vi "CompVisionUtil_EstimateFieldToRobot.vi"(4 "CameraToRobot":T1={"TRANSLATION"={"X"=0.0, "Y"=0.0}, "ROTATION"={"VALUE"=0.0, "COS"=1.0, "SIN"=0.0}, "xF"=FALSE} {"ROTATION"."SIN" format="%13.4f"; "ROTATION"."COS" format="%13.4f"; "ROTATION"."VALUE" format="%13.4f"; "TRANSLATION"."Y" format="%14.3f"; "TRANSLATION"."X" format="%14.3f"}, 5 "cameraHeight_Meters":dbl, 6 "FieldToTarget":T4={"TRANSLATION"={"X"=0.0, "Y"=0.0}, "ROTATION"={"VALUE"=0.0, "COS"=1.0, "SIN"=0.0}} {"ROTATION"."SIN" format="%13.4f"; "ROTATION"."COS" format="%13.4f"; "ROTATION"."VALUE" format="%13.4f"; "TRANSLATION"."Y" format="%14.3f"; "TRANSLATION"."X" format="%14.3f"}, 7 "targetHeight_Meters":dbl, 8 "GyroAngle":T3={"VALUE"=0.0, "COS"=1.0, "SIN"=0.0} {"SIN" format="%13.4f"; "COS" format="%13.4f"; "VALUE" format="%13.4f"}, 9 "TargetYaw":T3={"VALUE"=0.0, "COS"=1.0, "SIN"=0.0} {"SIN" format="%13.4f"; "COS" format="%13.4f"; "VALUE" format="%13.4f"}, 10 "targetPitch_Radians":dbl, 11 "cameraPitch_Radians":dbl) -> (3 "EstimateFieldToRobot":T4={"TRANSLATION"={"X"=0.0, "Y"=0.0}, "ROTATION"={"VALUE"=0.0, "COS"=1.0, "SIN"=0.0}} {"ROTATION"."SIN" format="%13.4f"; "ROTATION"."COS" format="%13.4f"; "ROTATION"."VALUE" format="%13.4f"; "TRANSLATION"."Y" format="%14.3f"; "TRANSLATION"."X" format="%14.3f"})   [LabVIEW 2019, in "Trajectory_Library.lvlib"]
doc: "Estimate the position of the robot in the field.\n\nInputs:\n - CameraHeightMeters The physical height of the camera off the floor in meters.\n - TargetHeightMeters The physical height of the target off the floor in meters. \n This should be the height of whatever is being targeted (i.e. if the targeting\n region is set to top, this should be the height of the top of the target).\n - CameraPitchRadians The pitch of the camera from the horizontal plane in \n radians. Positive values up.\n - TargetPitchRadians The pitch of the target in the camera's lens in radians. Positive\n values up.\n - TargetYaw The observed yaw of the target. Note that this *must* be \n CCW-positive, and Photon returns CW-positive.\n - GyroAngle The current robot gyro angle, likely from odometry.\n - FieldToTarget A Pose2d representing the target position in the field coordinate \n system.\n - CameraToRobot The position of the robot relative to the camera. If the camera \n was mounted 3 inches behind the \"origin\" (usually physical center) of the\n robot, this would be Transform2d (3 inches, 0 inches, 0 degrees).\n\nOutputs\n - EstimateFieldToRobot -- The position of the robot in the field."
uses:
  Trajectory_Library.lvlib
  TypeDef/POSE2D.ctl
  TypeDef/TRANSLATION2D.ctl
  TypeDef/ROTATION2D.ctl
  TypeDef/TRANSFORM2D.ctl
  CompVisionUtil_EstimateFieldToCamera.vi
  Pose2d_TransformBy.vi
  Transform2d_Create_TransRot.vi
  Rotation2d_UnaryMinus.vi
  Rotation2d_Minus.vi
  Pose2d_getRotation.vi
  Rotation2d_GetAngleCosSin.vi
  Transform2d_Inverse.vi
  Translation2d_RotateBy.vi
  Translation2d_Plus.vi
  Rotation2d_Plus.vi
  Pose2d_New_TRRO.vi
  Rotation2d_CreateAngle.vi
  Rotation2d_RotateBy.vi
  Translation2d_UnaryMinus.vi
  Translation2d_Create.vi
  Rotation2d_CreateXY.vi
  Util_CalcDist.vi
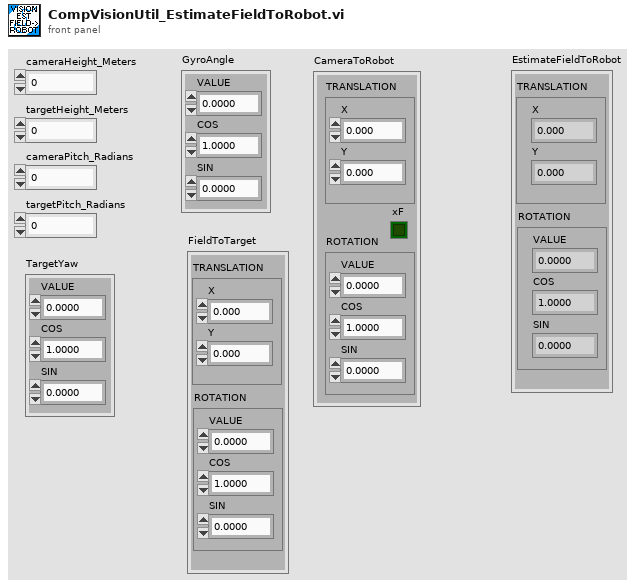
[diagram p1: front panel]
types:
  T1 = typedef "Trajectory_Library.lvlib/TRANSFORM2D.ctl" = cluster{"TRANSLATION":T2, "ROTATION":T3, "xF":bool}
  T2 = typedef "Trajectory_Library.lvlib/TRANSLATION2D.ctl" = cluster{"X":dbl, "Y":dbl}
  T3 = typedef "Trajectory_Library.lvlib/ROTATION2D.ctl" = cluster{"VALUE":dbl, "COS":dbl, "SIN":dbl}
  T4 = typedef "Trajectory_Library.lvlib/POSE2D.ctl" = cluster{"TRANSLATION":T2, "ROTATION":T3}
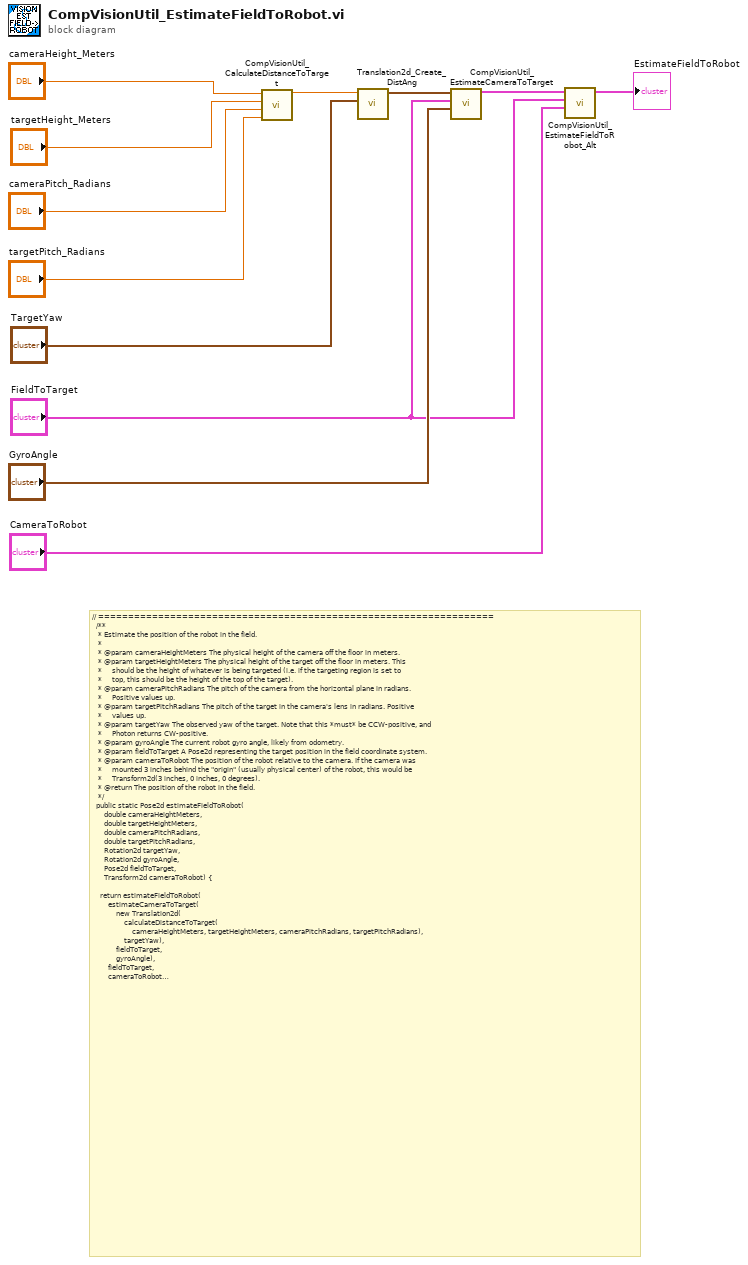
[diagram p0: block diagram]
diagram:
  # "// ==================================================================\n  /**\n   * Estimate the position of the robot in the field.\n   *\n   * @param cameraHeightMeters The physical height of the camera off the floor in meters.\n   * @param targetHeightMeters The physical height of the target off the floor in meters. This\n   *     should be the height of whatever is being targeted (i.e. if the targeting region is set to\n   *     top, this should be the height of the top of the target).\n   * @param cameraPitchRadians The pitch of the camera from the horizontal plane in radians.\n   *     Positive values up.\n   * @param targetPitchRadians The pitch of the target in the camera's lens in radians. Positive\n   *     values up.\n   * @param targetYaw The observed yaw of the target. Note that this *must* be CCW-positive, and\n   *     Photon returns CW-positive.\n   * @param gyroAngle The current robot gyro angle, likely from odometry.\n   * @param fieldToTarget A Pose2d representing the target position in the field coordinate system.\n   * @param cameraToRobot The position of the robot relative to the camera. If the camera was\n   *     mounted 3 inches behind the \"origin\" (usually physical center) of the robot, this would be\n   *     Transform2d(3 inches, 0 inches, 0 degrees).\n   * @return The position of the robot in the field.\n   */\n  public static Pose2d estimateFieldToRobot(\n      double cameraHeightMeters,\n      double targetHeightMeters,\n      double cameraPitchRadians,\n      double targetPitchRadians,\n      Rotation2d targetYaw,\n      Rotation2d gyroAngle,\n      Pose2d fieldToTarget,\n      Transform2d cameraToRobot) {\n\n    return estimateFieldToRobot(\n        estimateCameraToTarget(\n            new Translation2d(\n                calculateDistanceToTarget(\n                    cameraHeightMeters, targetHeightMeters, cameraPitchRadians, targetPitchRadians),\n                targetYaw),\n            fieldToTarget,\n            gyroAngle),\n        fieldToTarget,\n        cameraToRobot);\n  }"
  n1 = call "CompVisionUtil_CalculateDistanceToTarget.vi"("targetPitch_Radians"="targetPitch_Radians", "cameraPitch_Radians"="cameraPitch_Radians", "targetHeight_Meters"="targetHeight_Meters", "cameraHeight_Meters"="cameraHeight_Meters") -> ("DistanceToTarget_Meters"=w3:dbl)  [unwired: 7 in]
  n2 = call "Translation2d_Create_DistAng.vi"("Angle"="TargetYaw", "Dist"=w3) -> ("TRANSLATION"=w1:T2)  [unwired: 9 in]
  n3 = call "CompVisionUtil_EstimateCameraToTarget.vi"("GyroAngle"="GyroAngle", "FieldToTarget"="FieldToTarget", "CameraToTargetTranslation"=w1) -> ("EstimateCameraToTarget"=w10:T1)  [unwired: 8 in]
  n4 = call "CompVisionUtil_EstimateFieldToRobot_Alt.vi"("CameraToRobot"="CameraToRobot", "FieldToTarget"="FieldToTarget", "CameraToTarget"=w10) -> ("EstimatedFieldToRobot"=→"EstimateFieldToRobot":T4)  [unwired: 8 in]
